vi "Main.vi"() -> ()   [LabVIEW 2013]
doc: "Use this template to build a simple state machine design pattern. Each state executes code and determines which state to transition to."
uses:
  controls/State.ctl
  controls/ProjectState.ctl
  <instrlib>/IMS stepper motors/Address.ctl
  <instrlib>/Watlow EZ-ZONE/Public/Watlow_Set_Parameter.ctl
  <vilib>/Utility/file.llb/Read From Spreadsheet File (string).vi
  controls/Microprobe Vars.ctl
panel:
  in  "Tab Control":T1(tab)
  in  "Samples directory":path
  in  "Watlow channel":refnum<visa-resource-name>="COM3"
  in  "Sample name":string
  in  "Motor channel":refnum<visa-resource-name>="COM6"
  in  "MFC Channel":refnum<visa-resource-name>="COM5"
  in  "Active MFC address":i32=7
  in  "Inert MFC address":i32=8
  in  "ProbeTargetState":T2 {"Telem" format="%#.0f"; "GasC" format="%#_13g"; "GasB" format="%#_13g"; "GasA" format="%#_13g"; "Z" format="%.3g"; "Y" format="%.3g"; "X" format="%.3g"; "RampRate" format="%#_13g"}
  out "CurrentProbeState":T3 {"Tset" format="%#_13g"; "GasC" format="%.0g"; "GasB" format="%#_13g"; "GasA" format="%#_13g"; "Z" format="%#_13g"; "Y" format="%.3g"; "X" format="%.3g"; "RampRate" format="%.3g"}
  in  "Solenoid 1-3 open":bool=TRUE
  in  "Jog to X":dbl format="%.3g"
  in  "Jog to Y":dbl format="%.3g"
  in  "Jog":bool
  out "Microprobe state":T4
  out "Test sequence":string[][](table)
  out "Read program":bool
  out "Test sequence path":path
  out "Stop program":bool=TRUE
  out "Program state":T5
  in  "Exit":bool
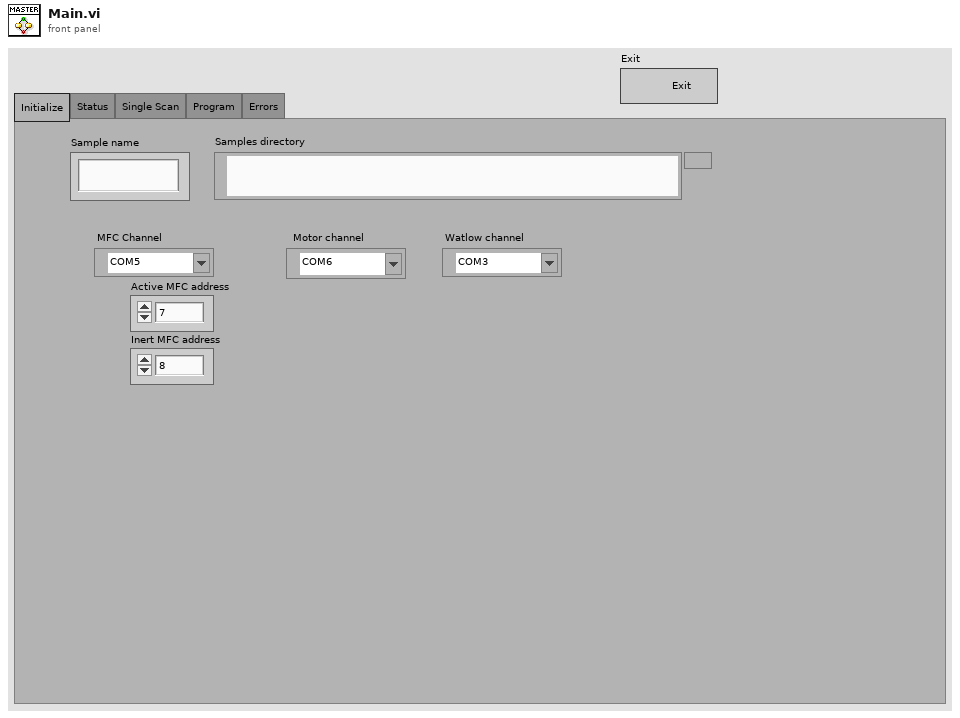
[diagram p1: front panel]
types:
  T1 = enum32{"Initialize", "Status", "Single Scan", "Program", "Errors"}
  T2 = typedef "Microprobe Vars.ctl" = cluster{"Telem":dbl, "RampRate":dbl, "X":dbl, "Y":dbl, "Z":dbl, "GasA":dbl, "GasB":dbl, "GasC":dbl, "Tset":dbl}
  T3 = typedef "Microprobe Vars.ctl" = cluster{"Telem":dbl, "Tset":dbl, "RampRate":dbl, "X":dbl, "Y":dbl, "Z":dbl, "GasA":dbl, "GasB":dbl, "GasC":dbl, "A-C\nopen":bool}
  T4 = typedef "State.ctl" = enum16{"Idle", "Jog", "Run AC Scan", "Run Program", "Exit"}
  T5 = typedef "ProjectState.ctl" = enum16{"Set gas", "Set temperature", "Move above position", "Wait for equilibrium", "Move to position", "Take measurement", "Write data to file", "Exit"}
  T6 = typedef "Address.ctl" = enum16{"X", "Y", "Z"}
  T7 = typedef "Watlow_Set_Parameter.ctl" = enum16{"Setpoint", "Ramp Rate", "Setpoint Min", "Setpoint Max"}
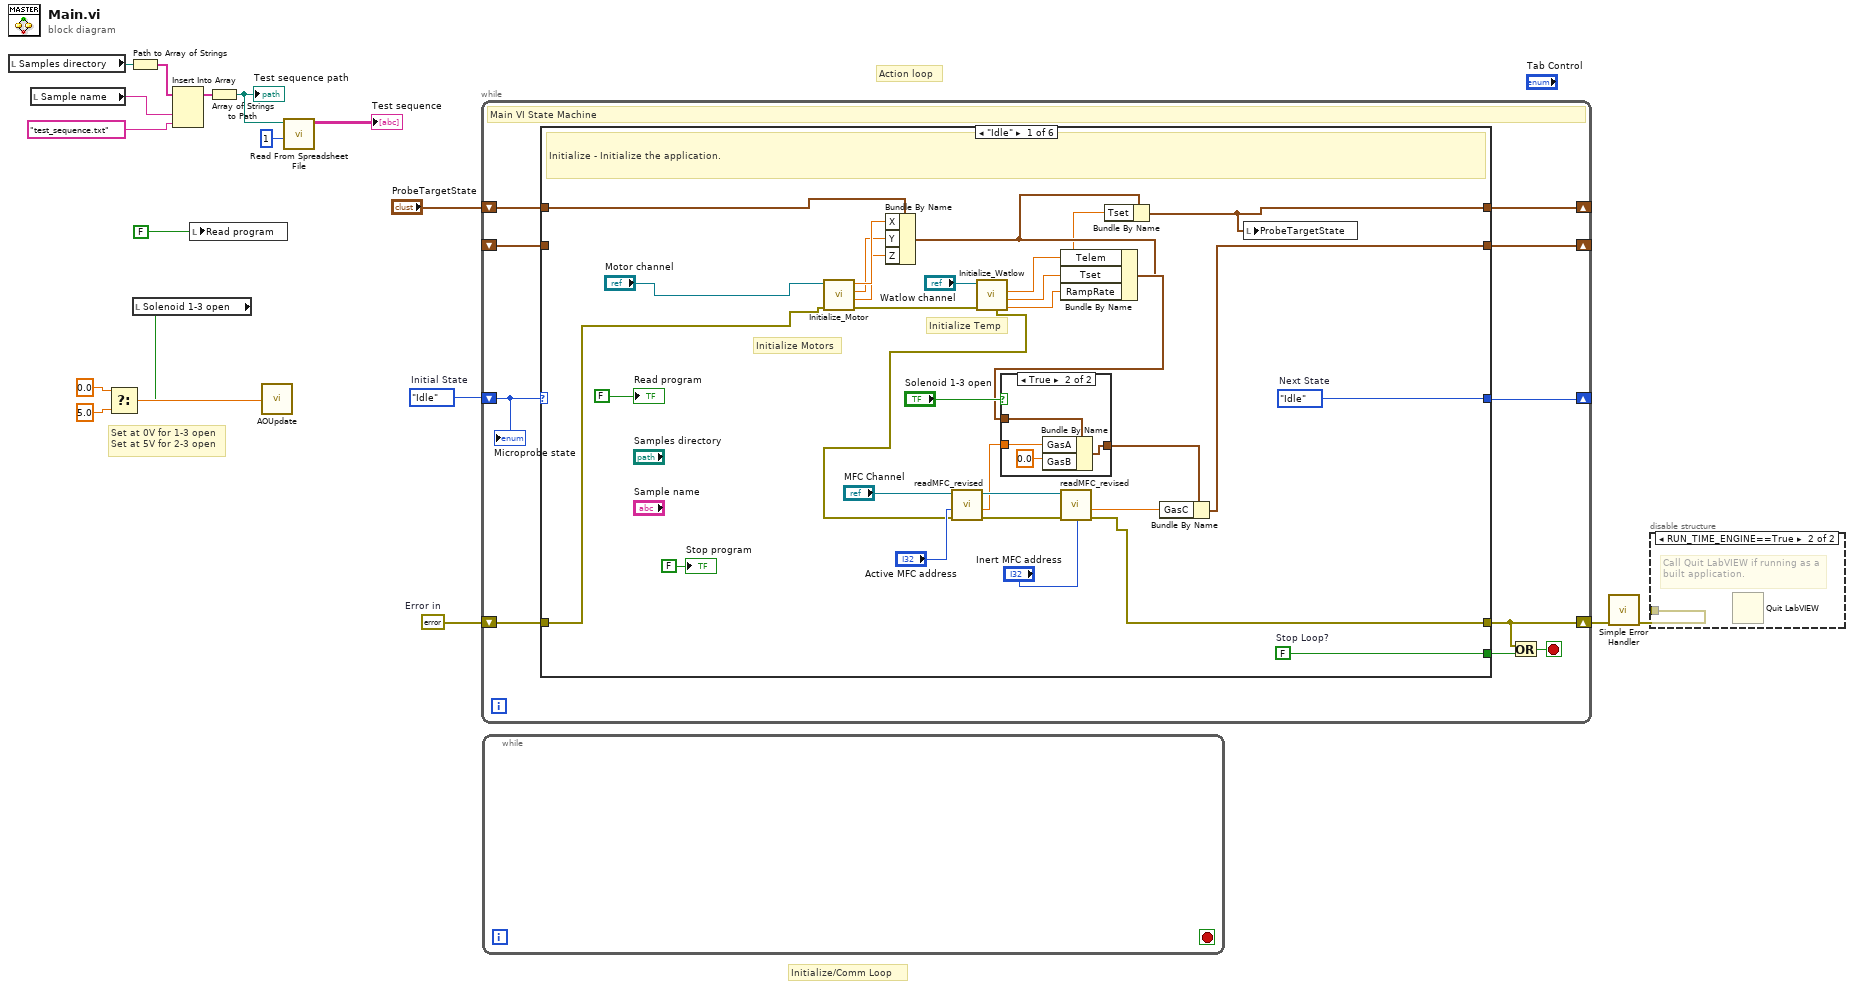
[diagram p0: block diagram]
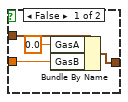
[diagram p3: hidden frame]
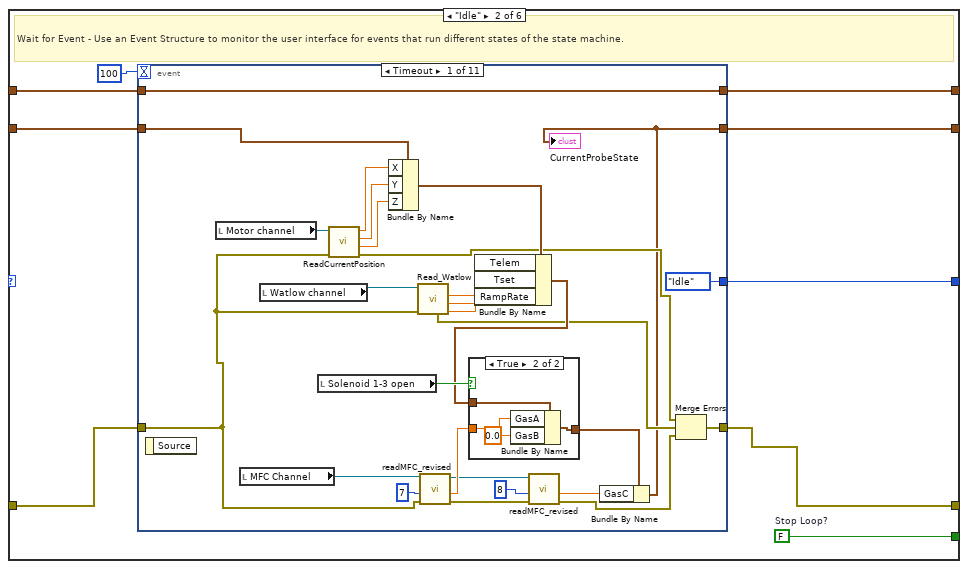
[diagram p4: hidden frame]
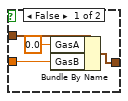
[diagram p5: hidden frame]
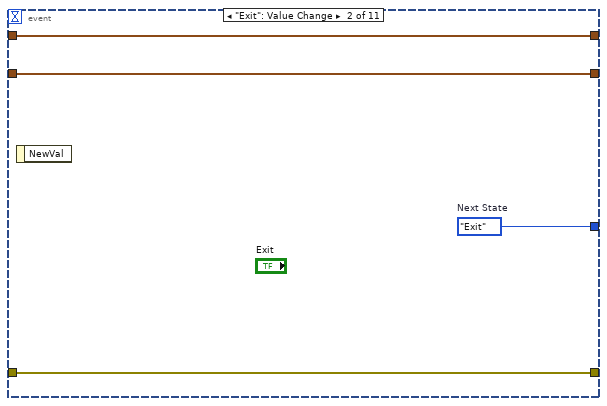
[diagram p6: hidden frame]
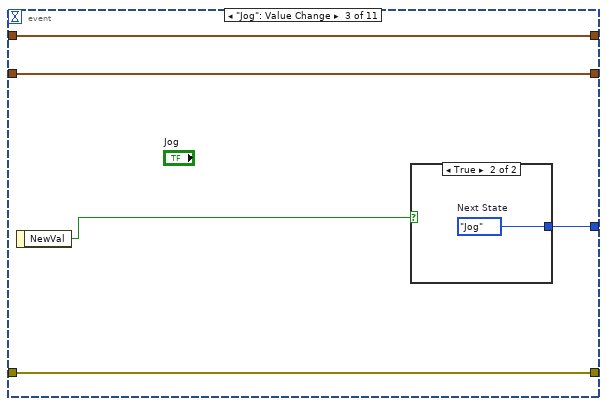
[diagram p7: hidden frame]
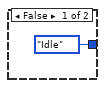
[diagram p8: hidden frame]
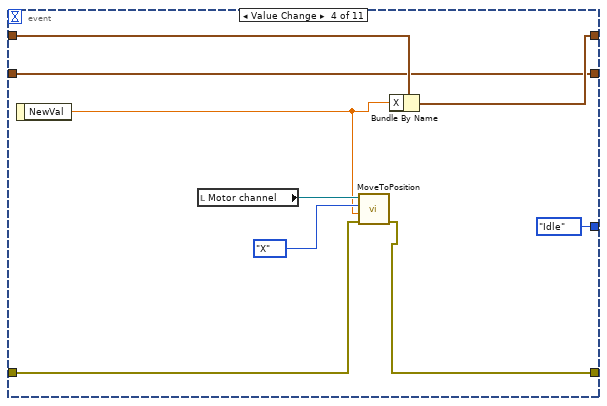
[diagram p9: hidden frame]
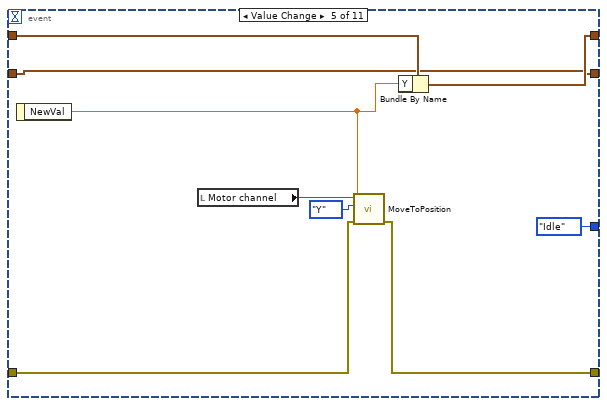
[diagram p10: hidden frame]
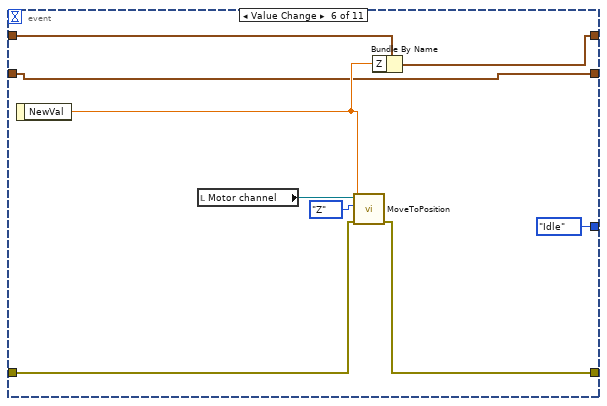
[diagram p11: hidden frame]
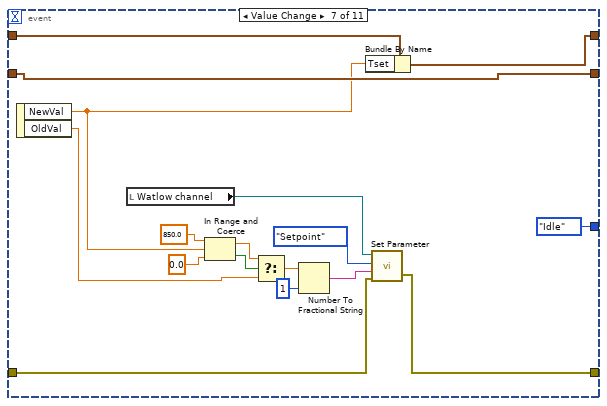
[diagram p12: hidden frame]
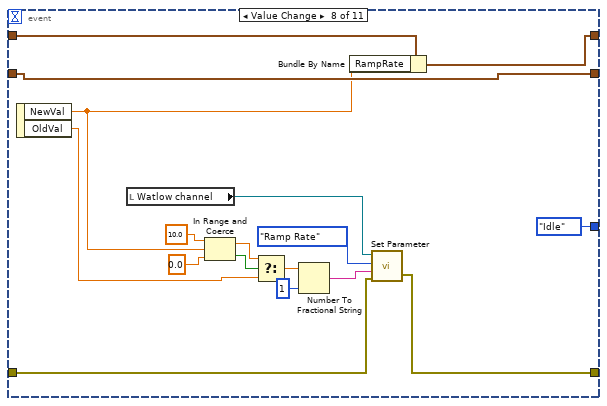
[diagram p13: hidden frame]
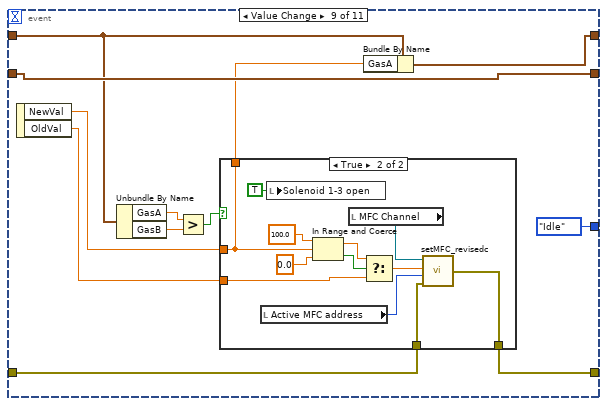
[diagram p14: hidden frame]
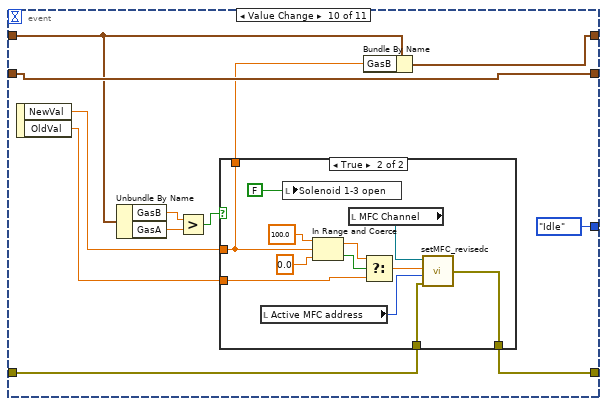
[diagram p16: hidden frame]
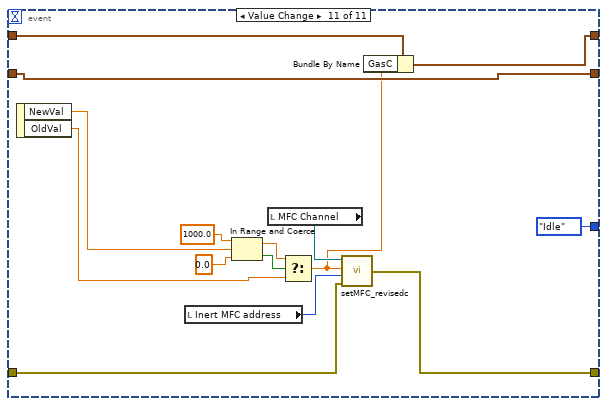
[diagram p18: hidden frame]
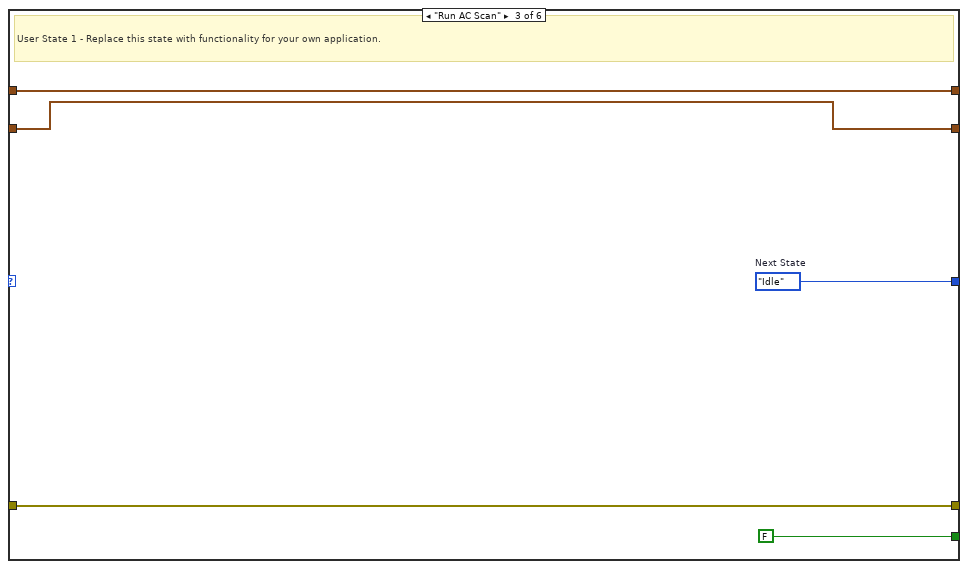
[diagram p19: hidden frame]
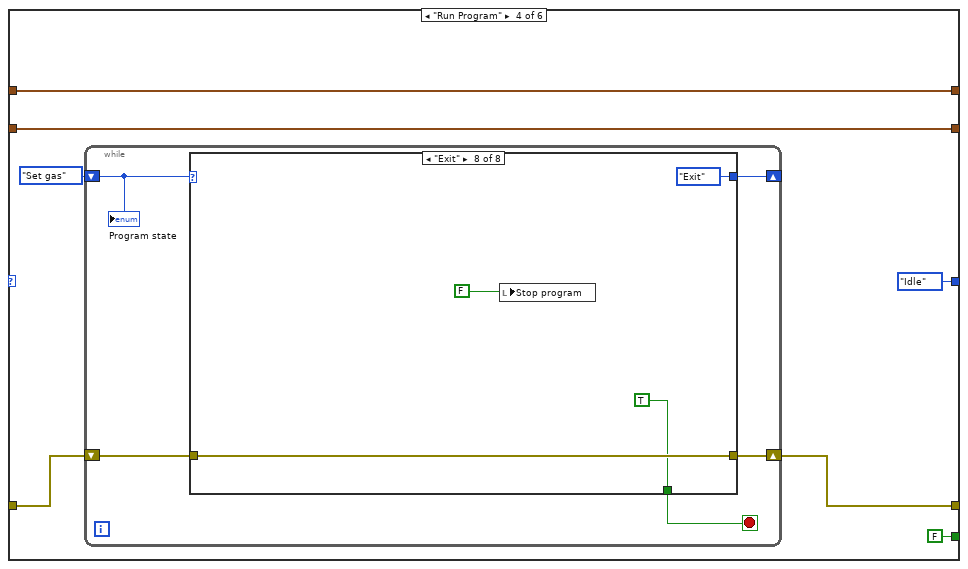
[diagram p20: hidden frame]
diagram:
  w17 = errorcluster {"status"=FALSE, "code"=0, "source"=""}  # Error in
  w18 = State."Idle"  # Initial State
  # "Set at 0V for 1-3 open\nSet at 5V for 2-3 open"
  # "Initialize/Comm Loop"
  # "Action loop"
  n1 = local read "Samples directory"() -> (w6:path)
  n2 = local read "Sample name"() -> (w8:string)
  n3 = Path to Array of Strings(0:w6) -> (2:w7:string[])  [unwired: 1 out]
  n4 = local read "Solenoid 1-3 open"() -> (w1:bool)
  n5 = Select(t=0.0, s=w1, f=5.0) -> (s? t:f=w4:dbl)
  n6 = Insert Into Array(array=w7, new element #1=w8, new element #2="test_sequence.txt") -> (w10:string[])  [unwired: 1 in]
  n7 = local write "Read program"(FALSE) -> ()
  n8 = Array of Strings to Path(0:w10) -> (2:w11:path)  [unwired: 1 in]
  "Test sequence path" <- w11
  n9 = call <vilib>:"AOUpdate.vi"("Analog Output 0 [volts]"=w4) -> ()  [unwired: 11 in, 4 out]
  n10 = call-poly <vilib>:"Read From Spreadsheet File.vi"("start of read offset (chars.:0)"=1, "file path (dialog if empty)"=w11) -> ("all rows"=→"Test sequence":string[][])  [unwired: 5 in, 4 out]
  n11 = while {
    shift-right: [w27] -> _
    shift-left: w18 -> [w28]
    shift-right: [w25] -> _
    shift-left: "ProbeTargetState" -> [w26]
    shift-right: [w19] -> w16
    shift-left: w17 -> [w24]
    shift-right: [w20] -> _
    shift-left: _ -> [w21]
    stop <- w22 stop-if-true
    # "Main VI State Machine"
    n12 = case shown="\"Idle\"" w28 {
      tunnel: [w58 w75 w255 State."Idle" ("(Value Not Used)") w327 w336] -> w27
      tunnel: [w57 w74 FALSE ("Stop Loop?") FALSE ("Stop Loop?") FALSE ("Stop Loop?") w334] -> w23
      tunnel: w26 -> [w54 w73 w253 w257 w326 w335]
      tunnel: [w31 w72 w253 w257 w316 w335] -> w25
      tunnel: w24 -> [w38 w71 w252 w261 w318 w332]
      tunnel: [w43 w70 w252 w260 w317 w330] -> w19
      tunnel: [w34 w68 w251 w258 w315 w333] -> w20
      tunnel: w21 -> [_ w67 w251 w258 w315 w333]
      frame "Idle" {
        w57 = FALSE  # Stop Loop?
        w58 = State."Idle"  # Next State
        # "Initialize Temp"
        # "Initialize Motors"
        # "Initialize - Initialize the application."
        n13 = call <instrlib>:"Initialize_Motor.vi"("error in"=w38, "Motor channel"="Motor channel") -> ("error out"=w55:errorcluster, "Z"=w51:dbl, "Y"=w52:dbl, "X"=w53:dbl)  [unwired: 6 in]
        n14 = Bundle By Name(cluster=w54, "X"=w53, "Y"=w52, "Z"=w51) -> (w33:T2)
        n15 = call <instrlib>:"Initialize_Watlow.vi"("Error In"=w55, "Watlow channel"="Watlow channel") -> ("Ramp rate"=w35:dbl, "Setpoint"=w32:dbl, "Current temp"=w36:dbl, "Error Out"=w49:errorcluster)  [unwired: 4 in, 1 out]
        n16 = call <instrlib>:"readMFC_revised.vi"("error in"=w49, "channel"="Active MFC address", "VISA resource name"="MFC Channel") -> ("error out"=w45:errorcluster, "flow rate sccm"=w40:dbl, "VISA resource name out"=w47:refnum<visa-resource-name>)  [unwired: 6 in]
        n17 = Bundle By Name(cluster=w33, "Telem"=w36, "Tset"=w32, "RampRate"=w35) -> (w41:T2)
        n18 = case shown="True" "Solenoid 1-3 open" {
          tunnel: w41 -> [w61 w66]
          tunnel: w40 -> [w62 w65]
          tunnel: [w60 w64] -> w39
          frame False {
            n19 = Bundle By Name(cluster=w61, "GasA"=0.0, "GasB"=w62) -> (w60:T2)
          }
          frame True {
            n20 = Bundle By Name(cluster=w66, "GasA"=w65, "GasB"=0.0) -> (w64:T2)
          }
        }
        n21 = call <instrlib>:"readMFC_revised.vi"("error in"=w45, "channel"="Inert MFC address", "VISA resource name"=w47) -> ("error out"=w43:errorcluster, "flow rate sccm"=w44:dbl)  [unwired: 6 in, 1 out]
        n22 = Bundle By Name(cluster=w33, "Tset"=w32) -> (w31:T2)
        n23 = Bundle By Name(cluster=w39, "GasC"=w44) -> (w34:T2)
        n24 = local write "ProbeTargetState"(w31) -> ()
        "Read program" <- FALSE ("Read program")
        "Stop program" <- FALSE ("Stop program")
      }
      frame "Idle" {
        w74 = FALSE  # Stop Loop?
        # "Wait for Event - Use an Event Structure to monitor the user interface for events that run different states of the state machine."
        n25 = event shown="[0] Timeout" {
          selector: _ -> [_ _ _ _ _ _ _ _ _ _ _]
          dyn-events: _ -> [_ _ _ _ _ _ _ _ _ _ _]
          timeout: 100 -> [_ _ _ _ _ _ _ _ _ _ _]
          tunnel: [State."Idle" ("Next State") w115 w120 State."Idle" ("Next State") State."Idle" ("Next State") State."Idle" ("Next State") State."Idle" ("Next State") State."Idle" ("Next State") State."Idle" ("Next State") State."Idle" ("Next State") State."Idle" ("Next State")] -> w75
          tunnel: w73 -> [w103 w114 w119 w127 w136 w145 w166 w183 w188 w214 w244]
          tunnel: [w103 w114 w119 w126 w135 w144 w165 w182 w195 w221 w250] -> w72
          tunnel: w71 -> [w78 w113 w118 w129 w139 w148 w151 w168 w190 w216 w246]
          tunnel: [w81 w113 w118 w128 w138 w147 w150 w167 w189 w215 w245] -> w70
          tunnel: [w76 w112 w117 w123 w132 w141 w163 w180 w193 w219 w248] -> w68
          tunnel: w67 -> [w83 w112 w117 w123 w132 w141 w163 w180 w193 w219 w248]
          event Timeout {
            n26 = event-data() -> ()  [unwired: 1 in, 1 out]
            n27 = local read "Motor channel"() -> (w84:refnum<visa-resource-name>)
            n28 = local read "MFC Channel"() -> (w100:refnum<visa-resource-name>)
            n29 = local read "Watlow channel"() -> (w88:refnum<visa-resource-name>)
            n30 = local read "Solenoid 1-3 open"() -> (w101:bool)
            n31 = call <instrlib>:"ReadCurrentPosition.vi"("error in"=w78, "Motor channel"=w84) -> ("error out"=w77:errorcluster, "Z"=w87:dbl, "Y"=w86:dbl, "X"=w85:dbl)  [unwired: 5 in, 1 out]
            n32 = Bundle By Name(cluster=w83, "X"=w85, "Y"=w86, "Z"=w87) -> (w90:T2)
            n33 = call <instrlib>:"Read_Watlow.vi"("Error In"=w78, "Watlow channel"=w88) -> ("Ramp rate"=w92:dbl, "Setpoint"=w91:dbl, "Current temp"=w89:dbl, "Error Out"=w79:errorcluster)  [unwired: 4 in, 1 out]
            n34 = call <instrlib>:"readMFC_revised.vi"("error in"=w78, "channel"=7, "VISA resource name"=w100) -> ("error out"=w96:errorcluster, "flow rate sccm"=w98:dbl, "VISA resource name out"=w94:refnum<visa-resource-name>)  [unwired: 6 in]
            n35 = Bundle By Name(cluster=w90, "Telem"=w89, "Tset"=w91, "RampRate"=w92) -> (w82:T2)
            n36 = case shown="True" w101 {
              tunnel: w82 -> [w106 w111]
              tunnel: w98 -> [w107 w110]
              tunnel: [w105 w109] -> w99
              frame False {
                n37 = Bundle By Name(cluster=w106, "GasA"=0.0, "GasB"=w107) -> (w105:T2)
              }
              frame True {
                n38 = Bundle By Name(cluster=w111, "GasA"=w110, "GasB"=0.0) -> (w109:T2)
              }
            }
            n39 = call <instrlib>:"readMFC_revised.vi"("error in"=w96, "channel"=8, "VISA resource name"=w94) -> ("error out"=w80:errorcluster, "flow rate sccm"=w97:dbl)  [unwired: 6 in, 1 out]
            n40 = Bundle By Name(cluster=w99, "GasC"=w97) -> (w76:T2)
            "CurrentProbeState" <- w76
            n41 = Merge Errors(w77, w79, w80) -> (w81:errorcluster)
          }
          event "Exit": Value Change {
            w115 = State."Exit"  # Next State
            n42 = event-data() -> ()  [unwired: 1 in, 1 out]
          }
          event "Jog": Value Change {
            n43 = event-data() -> ("NewVal"=w116:bool)  [unwired: 1 in]
            n44 = case shown="True" w116 {
              tunnel: [State."Idle" ("Next State") w122] -> w120
              frame False {
              }
              frame True {
                w122 = State."Jog"  # Next State
              }
            }
          }
          event Value Change {
            n45 = event-data() -> ("NewVal"=w125:dbl)  [unwired: 1 in]
            n46 = local read "Motor channel"() -> (w131:refnum<visa-resource-name>)
            n47 = call <instrlib>:"MoveToPosition.vi"("error out 2"=w129, "Position"=w125, "Address"=Address."X", "Motor channel"=w131) -> ("error out"=w128:errorcluster)  [unwired: 5 in, 2 out]
            n48 = Bundle By Name(cluster=w127, "X"=w125) -> (w126:T2)
          }
          event Value Change {
            n49 = event-data() -> ("NewVal"=w134:dbl)  [unwired: 1 in]
            n50 = local read "Motor channel"() -> (w140:refnum<visa-resource-name>)
            n51 = call <instrlib>:"MoveToPosition.vi"("error out 2"=w139, "Position"=w134, "Address"=Address."Y", "Motor channel"=w140) -> ("error out"=w138:errorcluster)  [unwired: 5 in, 2 out]
            n52 = Bundle By Name(cluster=w136, "Y"=w134) -> (w135:T2)
          }
          event Value Change {
            n53 = event-data() -> ("NewVal"=w143:dbl)  [unwired: 1 in]
            n54 = local read "Motor channel"() -> (w149:refnum<visa-resource-name>)
            n55 = call <instrlib>:"MoveToPosition.vi"("error out 2"=w148, "Position"=w143, "Address"=Address."Z", "Motor channel"=w149) -> ("error out"=w147:errorcluster)  [unwired: 5 in, 2 out]
            n56 = Bundle By Name(cluster=w145, "Z"=w143) -> (w144:T2)
          }
          event Value Change {
            n57 = event-data() -> ("NewVal"=w153:dbl, "OldVal"=w152:dbl)  [unwired: 1 in]
            n58 = local read "Watlow channel"() -> (w154:refnum<visa-resource-name>)
            n59 = In Range and Coerce(upper limit=850.0, x=w153, lower limit=0.0) -> (coerced(x)=w162:dbl, In Range?=w157:bool)
            n60 = Select(t=w162, s=w157, f=w152) -> (s? t:f=w161:dbl)
            n61 = Number To Fractional String(number=w161, precision (6)=i16 1) -> (F-format string=w160:string)  [unwired: 2 in]
            n62 = Bundle By Name(cluster=w166, "Tset"=w153) -> (w165:T2)
            n63 = call <instrlib>:"Set Parameter.vi"("Error In"=w151, "Set Parameter"=Watlow_Set_Parameter."Setpoint", "Write Value"=w160, "PC Comms Port"=w154) -> ("Error Out"=w150:errorcluster)  [unwired: 1 out]
          }
          event Value Change {
            n64 = event-data() -> ("NewVal"=w170:dbl, "OldVal"=w169:dbl)  [unwired: 1 in]
            n65 = local read "Watlow channel"() -> (w171:refnum<visa-resource-name>)
            n66 = In Range and Coerce(upper limit=10.0, x=w170, lower limit=0.0) -> (coerced(x)=w179:dbl, In Range?=w174:bool)
            n67 = Select(t=w179, s=w174, f=w169) -> (s? t:f=w178:dbl)
            n68 = Number To Fractional String(number=w178, precision (6)=i16 1) -> (F-format string=w177:string)  [unwired: 2 in]
            n69 = Bundle By Name(cluster=w183, "RampRate"=w170) -> (w182:T2)
            n70 = call <instrlib>:"Set Parameter.vi"("Error In"=w168, "Set Parameter"=Watlow_Set_Parameter."Ramp Rate", "Write Value"=w177, "PC Comms Port"=w171) -> ("Error Out"=w167:errorcluster)  [unwired: 1 out]
          }
          event Value Change {
            n71 = event-data() -> ("NewVal"=w192:dbl, "OldVal"=w191:dbl)  [unwired: 1 in]
            n72 = Unbundle By Name(w188) -> ("GasA"=w187:dbl, "GasB"=w186:dbl)
            n73 = Greater?(x=w187, y=w186) -> (0:w185:bool)
            n74 = case shown="True" w185 {
              tunnel: w192 -> [_ w199]
              tunnel: w191 -> [w197 w205]
              tunnel: w190 -> [w196 w202]
              tunnel: [w196 w201] -> w189
              tunnel: [w197 w199] -> w184
              frame False {
              }
              frame True {
                n75 = local read "Active MFC address"() -> (w200:i32)
                n76 = local write "Solenoid 1-3 open"(TRUE) -> ()
                n77 = In Range and Coerce(upper limit=100.0, x=w199, lower limit=0.0) -> (coerced(x)=w209:dbl, In Range?=w208:bool)
                n78 = local read "MFC Channel"() -> (w204:refnum<visa-resource-name>)
                n79 = Select(t=w209, s=w208, f=w205) -> (s? t:f=w203:dbl)
                n80 = call <instrlib>:"setMFC_revisedc.vi"("error in (no error)"=w202, "channel"=w200, "Set Flow Rate sccm"=w203, "VISA resource name"=w204) -> ("error out"=w201:errorcluster)
              }
            }
            n81 = Bundle By Name(cluster=w188, "GasA"=w184) -> (w195:T2)
          }
          event Value Change {
            n82 = event-data() -> ("NewVal"=w218:dbl, "OldVal"=w217:dbl)  [unwired: 1 in]
            n83 = Unbundle By Name(w214) -> ("GasB"=w213:dbl, "GasA"=w212:dbl)
            n84 = Greater?(x=w213, y=w212) -> (0:w211:bool)
            n85 = case shown="True" w211 {
              tunnel: w218 -> [_ w225]
              tunnel: w217 -> [w223 w231]
              tunnel: w216 -> [w222 w228]
              tunnel: [w222 w227] -> w215
              tunnel: [w223 w225] -> w210
              frame False {
              }
              frame True {
                n86 = local read "Active MFC address"() -> (w226:i32)
                n87 = local write "Solenoid 1-3 open"(FALSE) -> ()
                n88 = In Range and Coerce(upper limit=100.0, x=w225, lower limit=0.0) -> (coerced(x)=w235:dbl, In Range?=w234:bool)
                n89 = local read "MFC Channel"() -> (w230:refnum<visa-resource-name>)
                n90 = Select(t=w235, s=w234, f=w231) -> (s? t:f=w229:dbl)
                n91 = call <instrlib>:"setMFC_revisedc.vi"("error in (no error)"=w228, "channel"=w226, "Set Flow Rate sccm"=w229, "VISA resource name"=w230) -> ("error out"=w227:errorcluster)
              }
            }
            n92 = Bundle By Name(cluster=w214, "GasB"=w210) -> (w221:T2)
          }
          event Value Change {
            n93 = event-data() -> ("NewVal"=w243:dbl, "OldVal"=w247:dbl)  [unwired: 1 in]
            n94 = local read "Inert MFC address"() -> (w237:i32)
            n95 = In Range and Coerce(upper limit=1000.0, x=w243, lower limit=0.0) -> (coerced(x)=w242:dbl, In Range?=w241:bool)
            n96 = local read "MFC Channel"() -> (w238:refnum<visa-resource-name>)
            n97 = Select(t=w242, s=w241, f=w247) -> (s? t:f=w236:dbl)
            n98 = call <instrlib>:"setMFC_revisedc.vi"("error in (no error)"=w246, "channel"=w237, "Set Flow Rate sccm"=w236, "VISA resource name"=w238) -> ("error out"=w245:errorcluster)
            n99 = Bundle By Name(cluster=w244, "GasC"=w236) -> (w250:T2)
          }
        }
      }
      frame "Run AC Scan" {
        w255 = State."Idle"  # Next State
        # "User State 1 - Replace this state with functionality for your own application."
      }
      frame "Run Program" {
        n100 = while {
          shift-right: [w266] -> _
          shift-left: ProjectState."Set gas" ("Program state") -> [w267]
          shift-right: [w264] -> w260
          shift-left: w261 -> [w265]
          stop <- w263 stop-if-true
          n101 = case shown="\"Exit\"" w267 {
            tunnel: [w269 w275 w281 w287 w293 w299 w305 ProjectState."Exit" ("Program state 2")] -> w266
            tunnel: w265 -> [w271 w277 w283 w289 w295 w301 w307 w313]
            tunnel: [w271 w277 w283 w289 w295 w301 w307 w313] -> w264
            tunnel: [FALSE FALSE FALSE FALSE FALSE FALSE FALSE TRUE] -> w263
            frame "Set gas" {
              n102 = local read "Stop program"() -> (w270:bool)
              n103 = case shown="False" w270 {
                tunnel: [ProjectState."Exit" ("Program state 2") ProjectState."Set temperature" ("Program state 2")] -> w269
                frame False {
                }
                frame True {
                }
              }
            }
            frame "Set temperature" {
              n104 = local read "Stop program"() -> (w276:bool)
              n105 = case shown="True" w276 {
                tunnel: [ProjectState."Exit" ("Program state 2") ProjectState."Move above position" ("Program state 2")] -> w275
                frame False {
                }
                frame True {
                }
              }
            }
            frame "Move above position" {
              n106 = local read "Stop program"() -> (w282:bool)
              n107 = case shown="True" w282 {
                tunnel: [ProjectState."Exit" ("Program state 2") ProjectState."Wait for equilibrium" ("Program state 2")] -> w281
                frame False {
                }
                frame True {
                }
              }
            }
            frame "Wait for equilibrium" {
              n108 = local read "Stop program"() -> (w288:bool)
              n109 = case shown="True" w288 {
                tunnel: [ProjectState."Exit" ("Program state 2") ProjectState."Move to position" ("Program state 2")] -> w287
                frame False {
                }
                frame True {
                }
              }
            }
            frame "Move to position" {
              n110 = local read "Stop program"() -> (w294:bool)
              n111 = case shown="True" w294 {
                tunnel: [ProjectState."Exit" ("Program state 2") ProjectState."Take measurement" ("Program state 2")] -> w293
                frame False {
                }
                frame True {
                }
              }
            }
            frame "Take measurement" {
              n112 = local read "Stop program"() -> (w300:bool)
              n113 = case shown="True" w300 {
                tunnel: [ProjectState."Exit" ("Program state 2") ProjectState."Write data to file" ("Program state 2")] -> w299
                frame False {
                }
                frame True {
                }
              }
            }
            frame "Write data to file" {
              n114 = local read "Stop program"() -> (w306:bool)
              n115 = case shown="True" w306 {
                tunnel: [ProjectState."Exit" ("Program state 2") ProjectState."Exit" ("Program state 2")] -> w305
                frame False {
                }
                frame True {
                }
              }
            }
            frame "Exit" {
              n116 = local write "Stop program"(FALSE) -> ()
            }
          }
          "Program state" <- w267
        }
      }
      frame "Jog" {
        w327 = State."Idle"  # Next State
        # "User State 2 - Replace this state with functionality for your own application."
        n117 = local read "Motor channel"() -> (w322:refnum<visa-resource-name>)
        n118 = control-ref of="Y"() -> (w319:refnum<vi>)
        n119 = control-ref of="X"() -> (w320:refnum<vi>)
        n120 = control-ref of="RampRate"() -> (w321:refnum<vi>)
        n121 = Unbundle By Name(w315) -> ("Z"=w314:dbl)
        n122 = Bundle By Name(cluster=w326, "X"="Jog to X", "Y"="Jog to Y") -> (w316:T2)
        n123 = call <instrlib>:"JogToPosition.vi"("Target position refs"=w322, 1:w321, 2:w320, 3:w319, "Current position refs"="Jog to X", "Jog to X"="Jog to Y", "Jog to Y"=w314, "error out 2"=w318) -> ("error in 2"=w317:errorcluster)  [unwired: 7 in]
        n124 = local write "ProbeTargetState"(w316) -> ()
        n125 = case shown="No Error" w317 {
          frame No Error {
            n126 = local write "Jog"(FALSE) -> ()
          }
          frame Error {
          }
        }
      }
      frame "Exit" {
        w334 = TRUE  # Stop Loop?
        w336 = State."Exit"  # (Value Not Used)
        # "#CodeNeeded - Add any required cleanup code here."
        # "The state value is not used here since this is the last iteration of the state machine loop."
        # "Exit - Exit the application."
        n127 = call <instrlib>:"MDrive_Close_Com.vi"("error in"=w332) -> ("error out"=w331:errorcluster)  [unwired: 3 in]
        n128 = local read "Watlow channel"() -> (w329:refnum<visa-resource-name>)
        n129 = call <instrlib>:"EZZone_Close.vi"("PC Comms Port"=w329, "Error In"=w331) -> ("Error Out"=w330:errorcluster)  [unwired: 16 in, 1 out]
      }
    }
    n130 = Or(x=w19, y=w23) -> (x .or. y?=w22:bool)
    "Microprobe state" <- w28
  }
  n131 = while {
    stop <- _ stop-if-true
  }
  n132 = call <vilib>:"Simple Error Handler.vi"("error in (no error)"=w16) -> ("error out"=w15:errorcluster)  [unwired: 4 in, 4 out]
  n133 = disable-structure shown="RUN_TIME_ENGINE==True" {
    disable-tunnel: w15 -> [_ _]
    frame condition #0 (active) {
    }
    frame condition #1 {
      # "Call Quit LabVIEW if running as a built application."
      n134 = Quit LabVIEW() -> ()  [unwired: 1 in]
    }
  }
